vi "Profile Interpolation Custom Device.Async.vi"(10 "Parameters":variant, 11 "Process":refnum<class "Process.lvclass">) -> ()   [LabVIEW 2020, in "Profile Interpolation Engine.lvlib"]
uses:
  Profile Interpolation Engine.lvlib
  <vilib>/NI/NIVS Inline Async API/_VS Inline Async API/Process/Process.lvclass
  Shared/Types/Compiled.Settings.ctl
  <vilib>/NI VeriStand/Custom Device API/Custom Device Target Type.ctl
  <vilib>/NI/NIVS Inline Async API/_VS Inline Async API/Process/Process.lvclass/Process.ctl
  <vilib>/NI/NIVS Inline Async API/_VS Inline Async API/Process/Data Member Access/Read Data Access.vi
  <vilib>/NI/NIVS Inline Async API/_VS Inline Async API/Error Handling Process/SubVIs/Error.ConvertArray.vi
  Shared/SubVIs/Constants.vi
  <vilib>/NI/NIVS Inline Async API/_Data Access Engine/Data Access Engine/Methods/Write.Lookup.vi
  <vilib>/NI/NIVS Inline Async API/_Data Access Engine/Data Access Engine/Methods/Read.Lookup.vi
  <vilib>/NI/NIVS Inline Async API/_Data Access Engine/Data Access Engine/Data Access Engine.lvclass
  Shared/Profile Interpolation Shared.lvlib
  <vilib>/NI VeriStand/Custom Device API/Custom Device API.lvlib
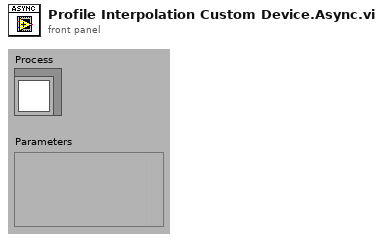
[diagram p1: front panel]
types:
  T1 = typedef "Profile Interpolation Shared.lvlib/Compiled.Settings.ctl" = cluster{"Name":string, "Create Limit Channels?":bool, "Profiles []":cluster{"Profile":dbl[][]}[], "Target.Type":T2}
  T2 = typedef "Custom Device API.lvlib/Custom Device Target Type.ctl" = enum16{"PharLap", "VxWorks", "Windows", "Linux_32_ARM", "Linux_x64"}
  T3 = typedef "Data Access Engine.lvlib/Data Access Engine.lvclass/Write.DVR.ctl" = refnum<data-value>
  T4 = typedef "Data Access Engine.lvlib/Data Access Engine.lvclass/Read.DVR.ctl" = refnum<data-value>
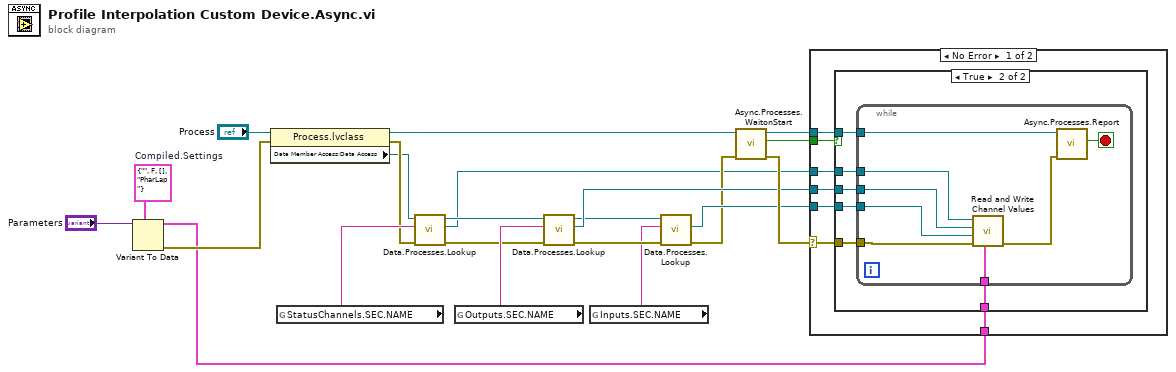
[diagram p0: block diagram]
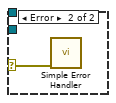
[diagram p3: hidden frame]
diagram:
  w3 = T1 {"Name"="", "Create Limit Channels?"=FALSE, "Profiles []"=[], "Target.Type"=enum."PharLap"}  # Compiled.Settings
  n1 = Variant To Data(type=w3, Variant="Parameters") -> (data=w1:T1, error out=w2:errorcluster)  [unwired: 1 in]
  n2 = property class="Process.lvclass"(reference="Process", error in=w2) -> (reference out=w13:refnum<class "Process.lvclass">, error out=w9:errorcluster, "Data Member Access:Data Access"=w7:refnum<class "Data Access Engine.lvclass">)
  n3 = global read "Constants.vi" "StatusChannels.SEC.NAME"() -> (w10:string)
  n4 = call-poly <vilib>:"Data.Processes.Lookup.vi"("error in (no error)"=w9, "Name"=w10, "Data Access API in"=w7) -> ("error out"=w8:errorcluster, "Ref"=w5:T3, "Data Access API out"=w6:refnum<class "Data Access Engine.lvclass">)  [unwired: 5 in, 1 out]
  n5 = global read "Constants.vi" "Outputs.SEC.NAME"() -> (w12:string)
  n6 = call-poly <vilib>:"Data.Processes.Lookup.vi"("error in (no error)"=w8, "Name"=w12, "Data Access API in"=w6) -> ("error out"=w18:errorcluster, "Ref"=w17:T3, "Data Access API out"=w16:refnum<class "Data Access Engine.lvclass">)  [unwired: 5 in, 1 out]
  n7 = global read "Constants.vi" "Inputs.SEC.NAME"() -> (w11:string)
  n8 = call-poly <vilib>:"Data.Processes.Lookup.vi"("error in (no error)"=w18, "Name"=w11, "Data Access API in"=w16) -> ("error out"=w15:errorcluster, "Ref"=w19:T4)  [unwired: 5 in, 2 out]
  n9 = call <vilib>:"Async.Processes.WaitonStart.vi"("error in (no error)"=w15, "Process"=w13) -> ("error out"=w20:errorcluster, "Execute"=w22:bool, "Process out"=w21:refnum<class "Process.lvclass">)  [unwired: 7 in]
  n10 = case shown="No Error" w20 {
    selector: w20 -> [w25 w44]
    tunnel: w22 -> [w29 _]
    tunnel: w21 -> [w28 _]
    tunnel: w17 -> [w27 _]
    tunnel: w19 -> [w26 _]
    tunnel: w5 -> [w24 _]
    tunnel: w1 -> [w23 _]
    frame No Error {
      n11 = case shown="True" w29 {
        tunnel: w25 -> [_ w32]
        tunnel: w28 -> [_ w33]
        tunnel: w26 -> [_ w35]
        tunnel: w27 -> [_ w34]
        tunnel: w24 -> [_ w31]
        tunnel: w23 -> [_ w30]
        frame False {
        }
        frame True {
          n12 = while {
            tunnel: w32 -> [w40]
            tunnel: w33 -> [w43]
            tunnel: w35 -> [w41]
            tunnel: w34 -> [w37]
            tunnel: w31 -> [w38]
            tunnel: w30 -> [w36]
            stop <- w42 stop-if-true
            n13 = call "Read and Write Channel Values.vi"("Compiled.Settings"=w36, "error in"=w40, "Inputs Reference in"=w41, "Outputs Reference in"=w37, "Status Reference in"=w38) -> ("error out"=w39:errorcluster)  [unwired: 6 in]
            n14 = call <vilib>:"Async.Processes.Report.vi"("Error"=w39, "Process in"=w43) -> ("Stop"=w42:bool)  [unwired: 8 in, 1 out]
          }
        }
      }
    }
    frame Error {
      n15 = call <vilib>:"Simple Error Handler.vi"("error in (no error)"=w44) -> ()  [unwired: 4 in, 5 out]
    }
  }
